vi "Write Addresses.vi"(0 "Address File":path) -> ()   [LabVIEW 2009]
uses:
  Message Address Global.vi
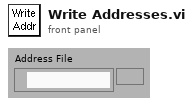
[diagram p1: front panel]
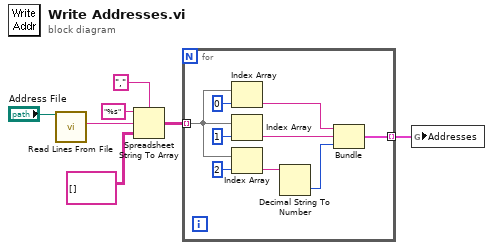
[diagram p0: block diagram]
diagram:
  n1 = call <vilib>:"Read Lines From File.vi"("file path (dialog if empty)"="Address File") -> ("line string"=w6:string)  [unwired: 5 in, 3 out]
  n2 = Spreadsheet String To Array(delimiter (Tab)=",", format string="%s", spreadsheet string=w6, array type (2D Dbl)=string[][] [] ("Array Constant")) -> (array=w2:string[][])
  n3 = for {
    tunnel: w2 -> [w16] mode=indexing
    tunnel: [w8] -> w1 mode=indexing
    n4 = Index Array(array=w16, index=0 ("Index")) -> (element=w9:string)
    n5 = Index Array(array=w16, index=1 ("Index")) -> (element=w10:string)
    n6 = Index Array(array=w16, index=2 ("Index")) -> (element=w12:string)
    n7 = Decimal String To Number(string=w12) -> (number=w11:i32)  [unwired: 2 in, 1 out]
    n8 = Bundle(w9, w10, w11) -> (w8:cluster{string, string, i32})  [unwired: 1 in]
  }
  n9 = global write "Message Address Global.vi" "Addresses"(w1) -> ()
